vi "MGI RWA Unreplace Characters.vi"(0 "String In":string) -> (2 "String Out":string)   [LabVIEW 2018]
doc: "This VI was created for use with the Read/Write Anything VIs. It converts any carriage return or line feed unique identifier strings in the string to carriage return and line feed characters.\n\nAuthored by Robert C. Mortensen\nsupport@mooregoodideas.com\nwww.mooregoodideas.com\n\nCopyright (c) 2010, Moore Good Ideas, Inc.\n\nAll rights reserved.\n\nRedistribution and use in source and binary forms, with or without modification, are permitted provided that the following conditions are met:\n\n * Redistributions of source code must retain the above copyright notice, this list of conditions and the following disclaimer.\n * Redistributions in binary form must reproduce the above copyright notice, this list of conditions and the following disclaimer in the documentation and/or other materials provided with the distribution.\n * Neither the name of Moore Good Ideas, Inc. nor the names of its contributors may be used to endorse or promote products derived from this software without specific prior written permission.\n\nTHIS SOFTWARE IS PROVIDED BY THE COPYRIGHT HOLDERS AND CONTRIBUTORS \"AS IS\" AND ANY EXPRESS OR IMPLIED WARRANTIES, INCLUDING, BUT NOT LIMITED TO, THE IMPLIED WARRANTIES OF MERCHANTABILITY AND FITNESS FOR A PARTICULAR PURPOSE ARE DISCLAIMED. IN NO EVENT SHALL THE COPYRIGHT OWNER OR CONTRIBUTORS BE LIABLE FOR ANY DIRECT, INDIRECT, INCIDENTAL, SPECIAL, EXEMPLARY, OR CONSEQUENTIAL DAMAGES (INCLUDING, BUT NOT LIMITED TO, PROCUREMENT OF SUBSTITUTE GOODS OR SERVICES; LOSS OF USE, DATA, OR PROFITS; OR BUSINESS INTERRUPTION) HOWEVER CAUSED AND ON ANY THEORY OF LIABILITY, WHETHER IN CONTRACT, STRICT LIABILITY, OR TORT (INCLUDING NEGLIGENCE OR OTHERWISE) ARISING IN ANY WAY OUT OF THE USE OF THIS SOFTWARE, EVEN IF ADVISED OF THE POSSIBILITY OF SUCH DAMAGE."
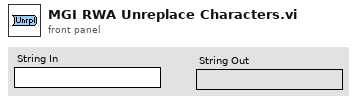
[diagram p1: front panel]
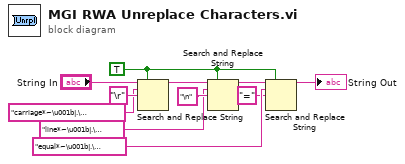
[diagram p0: block diagram]
diagram:
  w3 = TRUE ("replace all? (F)")
  n1 = Search and Replace String(replace all?=w3, input string="String In", search string="carriage*~\u001b|.\u0017return", replace string="\r" ("replace string (\"\")")) -> (result string=w9:string)  [unwired: 4 in, 3 out]
  n2 = Search and Replace String(replace all?=w3, input string=w9, search string="line*~\u001b|.\u0017feed", replace string="\n" ("replace string (\"\")")) -> (result string=w5:string)  [unwired: 4 in, 3 out]
  n3 = Search and Replace String(replace all?=w3, input string=w5, search string="equal*~\u001b|.\u0017sign", replace string="=" ("replace string (\"\")")) -> (result string=→"String Out":string)  [unwired: 4 in, 3 out]
